vi "Pulse - Build Wave.vi"(8 "error in (no error)":errorcluster, 10 "Channel List String":string, 11 "3300 in":refnum<class "3300.lvclass">) -> (0 "error out":errorcluster, 3 "3300 out":refnum<class "3300.lvclass">)   [LabVIEW 2019, in "3300.lvlib" / "3300.lvclass"]
uses:
  Library/3300.lvclass
  Library/3300.lvclass/3300.ctl
  Accessors/Write Local Resource.vi
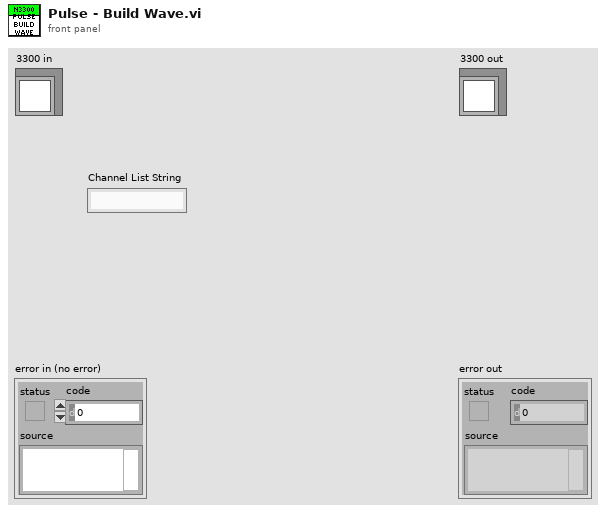
[diagram p1: front panel]
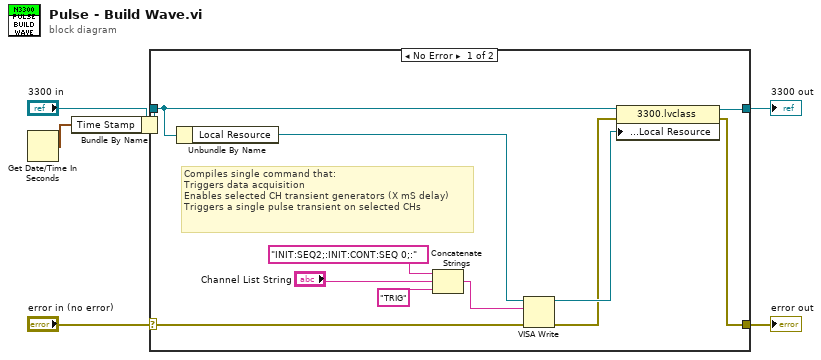
[diagram p0: block diagram]
diagram:
  n1 = Get Date/Time In Seconds() -> (seconds since 1Jan1904=w1:timestamp)
  n2 = Bundle By Name(cluster="3300 in", "Time Stamp"=w1) -> (w2:refnum<class "3300.lvclass">)
  n3 = case shown="No Error" "error in (no error)" {
    selector: "error in (no error)" -> [w13 w19]
    tunnel: [w7 w19] -> w5
    tunnel: [w12 w18] -> w3
    tunnel: w2 -> [w11 w18]
    frame No Error {
      # "Compiles single command that: \nTriggers data acquisition\nEnables selected CH transient generators (X mS delay)\nTriggers a single pulse transient on selected CHs"
      n4 = Unbundle By Name(w11) -> ("Local Resource"=w10:refnum<visa-resource-name>)
      n5 = Concatenate Strings("INIT:SEQ2;:INIT:CONT:SEQ 0;:" ("string"), "Channel List String", "TRIG" ("string")) -> (w17:string)
      n6 = VISA Write(VISA resource name=w10, write buffer=w17, error in (no error)=w13) -> (VISA resource name out=w9:refnum<visa-resource-name>, error out=w8:errorcluster)  [unwired: 1 out]
      n7 = property class="3300.lvclass"(reference=w11, error in=w8, "Private:Accessors:Local Resource"=w9) -> (reference out=w12:refnum<class "3300.lvclass">, error out=w7:errorcluster)
    }
    frame Error {
    }
  }
  "error out" <- w5
  "3300 out" <- w3
